vi "06.1 Injecting Errors.vi"() -> ()   [LabVIEW 2019]
uses:
  Support Files/02.4 DAQmx Configuration Cluster.ctl
  Support Files/03.2 States.ctl
  Support Files/03.2 State Machine Data.ctl
  <vilib>/DAQmx/write.llb/DAQmx Write (Analog DBL 1Chan 1Samp).vi
  <vilib>/Utility/file.llb/Write Delimited Spreadsheet (string).vi
  <vilib>/Utility/file.llb/Write Delimited Spreadsheet (DBL).vi
  <vilib>/DAQmx/create/channels.llb/DAQmx Create Channel (AO-Voltage-Basic).vi
  <vilib>/DAQmx/miscellaneous.llb/DAQmx Fill In Error Info.vi
panel:
  in  "DAQmx Configuration Cluster":T1={"Desired Sample Rate (Hz)"=-1.0, "sample mode"=10178, "Minimum value"=-1.0, "Maximum value"=-1.0, "Physical Channel"="", "units"=10143, "thermocouple type"=10072, "Samples per Channel"=0} {"thermocouple type" items=["J"=10072, "K"=10073, "N"=10077, "R"=10082, "S"=10085, "T"=10086, "B"=10047, "E"=10055]; "units" items=["Deg C"=10143, "Deg F"=10144, "Kelvins"=10325, "Deg R"=10145, "From Custom Scale"=10065]; "sample mode" items=["Finite Samples"=10178, "Continuous Samples"=10123, "Hardware Timed Single Point"=12522]}
  in  "Threshold (RMS)":dbl
  in  "Generate Stimulus":bool
  in  "Stop":bool
  in  "Clear":bool
  in  "Acquire":bool
  out "Graph":dbl[][](graph)
  out "Thershold Exceeded?":bool
  out "RMS Result per Channel":dbl[](array[numeric])
  # "ANALYSIS"
  # "EVENTS"
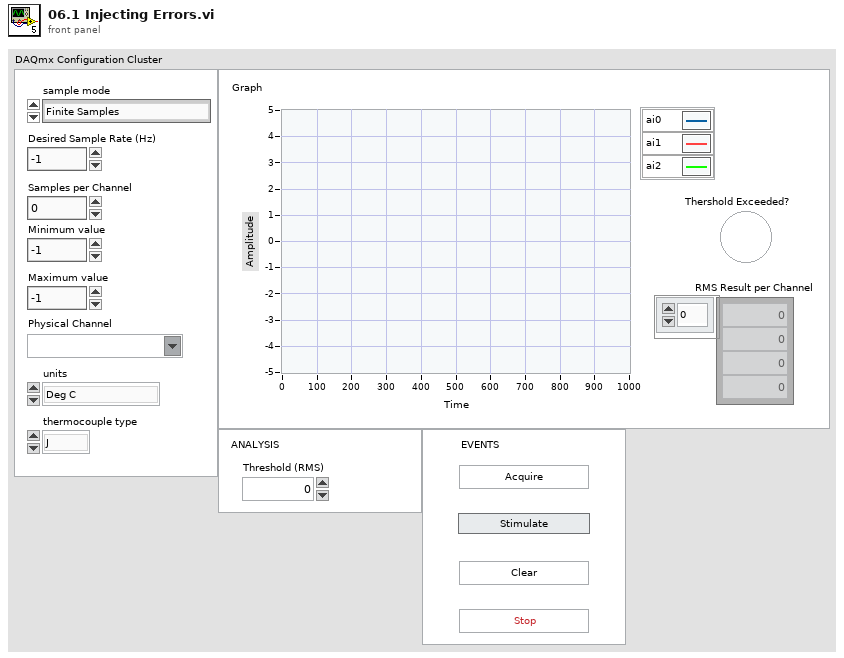
[diagram p1: front panel]
types:
  T1 = typedef "02.4 DAQmx Configuration Cluster.ctl" = cluster{"Desired Sample Rate (Hz)":dbl, "sample mode":i32, "Minimum value":dbl, "Maximum value":dbl, "Physical Channel":tag, "units":i32, "thermocouple type":i32, "Samples per Channel":i32}
  T2 = typedef "03.2 State Machine Data.ctl" = cluster{"Acquisition Data":dbl[][], "Stimulus?":bool}
  T3 = typedef "03.2 States.ctl" = enum16{"Initialize", "Update UI", "Update Stimulus", "Wait for event", "Acquire", "Analyze", "Log", "Clear", "Shutdown"}
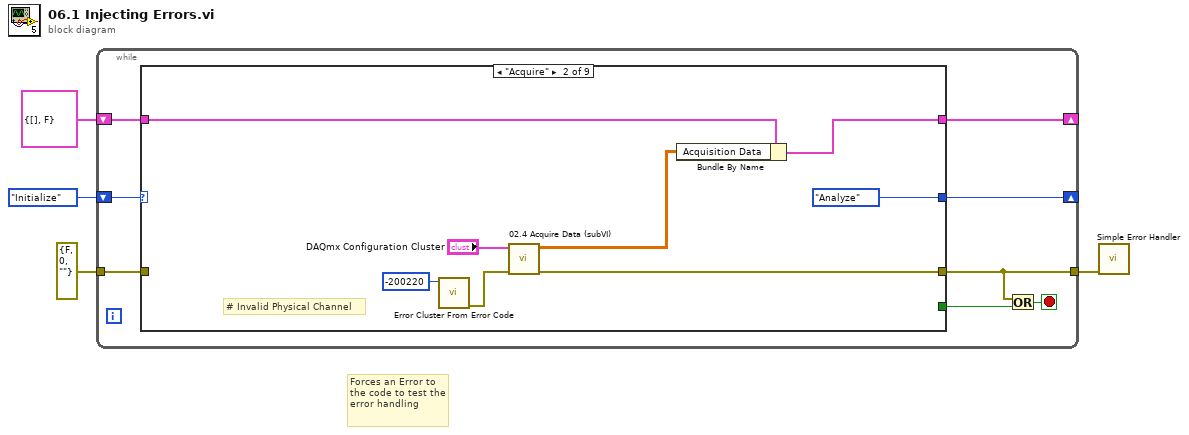
[diagram p0: block diagram]
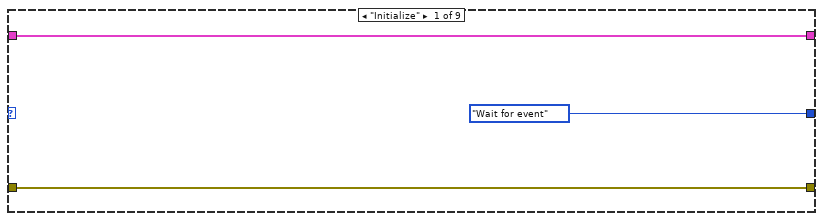
[diagram p2: hidden frame]
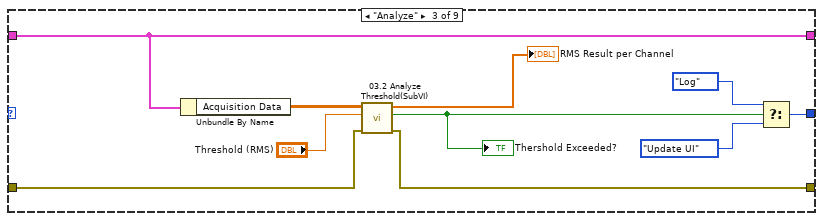
[diagram p3: hidden frame]
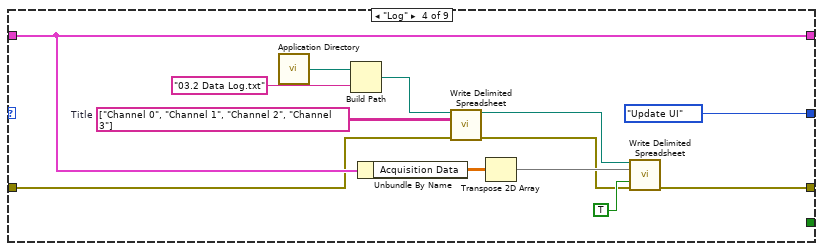
[diagram p4: hidden frame]
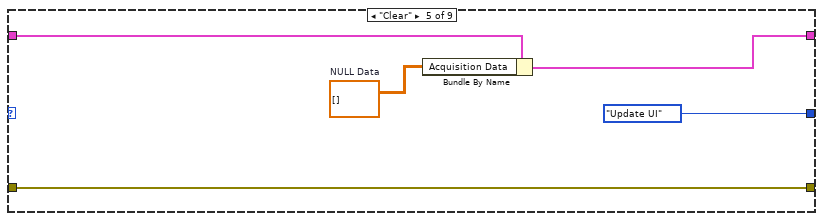
[diagram p5: hidden frame]
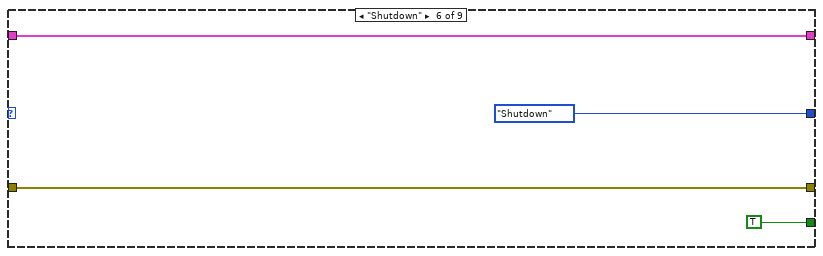
[diagram p6: hidden frame]
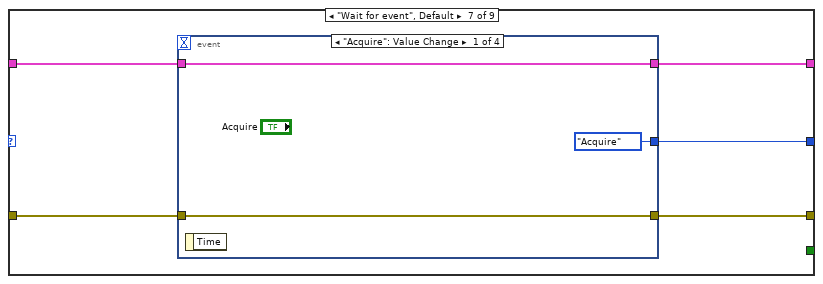
[diagram p7: hidden frame]
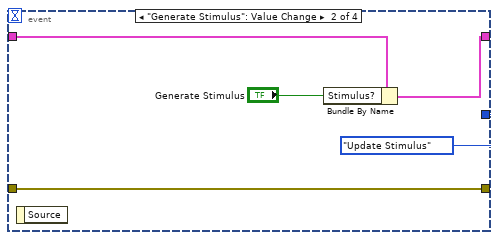
[diagram p8: hidden frame]
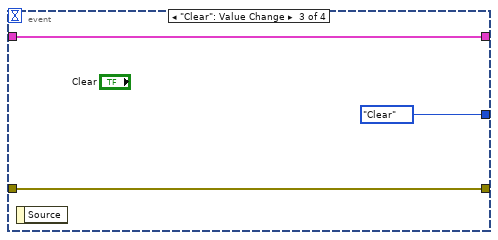
[diagram p9: hidden frame]
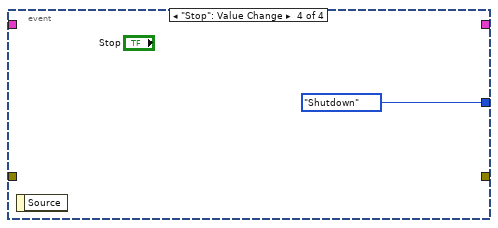
[diagram p10: hidden frame]
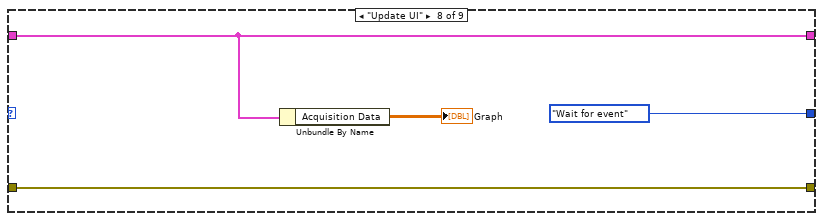
[diagram p11: hidden frame]
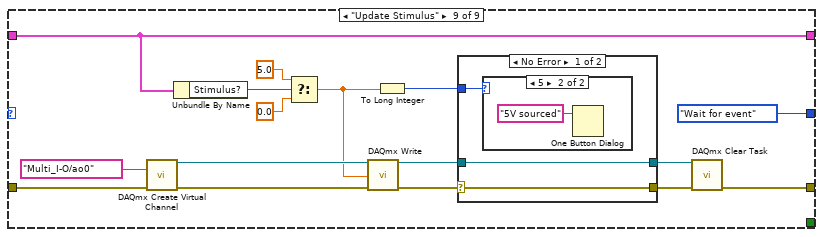
[diagram p12: hidden frame]
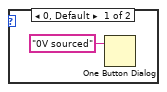
[diagram p13: hidden frame]
diagram:
  # "Forces an Error to the code to test the error handling"
  n1 = while {
    shift-right: [w11] -> _
    shift-left: 03.2_States."Initialize" ("State") -> [w12]
    tunnel: errorcluster {"status"=FALSE, "code"=0, "source"=""} ("error constant") -> [w10]
    tunnel: [w8] -> w2
    shift-right: [w7] -> _
    shift-left: T2 {"Acquisition Data"=[], "Stimulus?"=FALSE} -> [w6]
    stop <- w9 stop-if-true
    n2 = case shown="\"Acquire\"" w12 {
      tunnel: [03.2_States."Wait for event" ("State") 03.2_States."Analyze" ("State") w32 03.2_States."Update UI" ("State") 03.2_States."Update UI" ("State") 03.2_States."Shutdown" ("State") w60 03.2_States."Wait for event" ("State") 03.2_States."Wait for event" ("State")] -> w11
      tunnel: [w14 w20 w27 w44 w47 w53 w59 w74 w81] -> w8
      tunnel: w10 -> [w14 _ w28 w34 w47 w53 w58 w74 w92]
      tunnel: [w15 w22 w26 w42 w50 w54 w57 w76 w78] -> w7
      tunnel: w6 -> [w15 w23 w26 w42 w51 w54 w56 w76 w78]
      tunnel: [_ _ _ _ _ TRUE _ _ _] -> w5
      frame "Initialize" {
      }
      frame "Acquire" {
        # "# Invalid Physical Channel"
        n3 = call <vilib>:"Error Cluster From Error Code.vi"("error code (0)"=-200220) -> ("error out"=w17:errorcluster)  [unwired: 8 in]
        n4 = call "02.4 Acquire Data (subVI).vi"("Error In"=w17, "DAQmx Configuration Cluster"="DAQmx Configuration Cluster") -> ("error out"=w20:errorcluster, "2D DBL"=w21:dbl[][])  [unwired: 8 in]
        n5 = Bundle By Name(cluster=w23, "Acquisition Data"=w21) -> (w22:T2)
      }
      frame "Analyze" {
        n6 = Unbundle By Name(w26) -> ("Acquisition Data"=w33:dbl[][])
        n7 = call "03.2 Analyze Threshold(SubVI).vi"("Error In"=w28, "Threshold (RMS)"="Threshold (RMS)", "Data"=w33) -> ("Error Out"=w27:errorcluster, "Threshold exceeded?"=w29:bool, "RMS Results per Channel"=→"RMS Result per Channel":dbl[])  [unwired: 6 in]
        "Thershold Exceeded?" <- w29
        n8 = Select(t=03.2_States."Log" ("State"), s=w29, f=03.2_States."Update UI" ("State")) -> (s? t:f=w32:T3)
      }
      frame "Log" {
        w36 = string[][] [["Channel 0", "Channel 1", "Channel 2", "Channel 3"]]  # Title
        n9 = call <vilib>:"Application Directory.vi"() -> ("Application Directory"=w46:path)
        n10 = Build Path(base path=w46, name or relative path="03.2 Data Log.txt") -> (appended path=w37:path)
        n11 = Unbundle By Name(w42) -> ("Acquisition Data"=w41:dbl[][])
        n12 = call-poly <vilib>:"Write Delimited Spreadsheet.vi"("file path (dialog if empty)"=w37, "2D data"=w36, "error in (no error)"=w34) -> ("new file path (Not A Path if cancelled)"=w39:path, "error out"=w35:errorcluster)  [unwired: 11 in]
        n13 = Transpose 2D Array(2D array=w41) -> (transposed array=w40:dbl[][])
        n14 = call-poly <vilib>:"Write Delimited Spreadsheet.vi"("file path (dialog if empty)"=w39, "2D data"=w40, "append to file? (new file:F)"=TRUE, "error in (no error)"=w35) -> ("error out"=w44:errorcluster)  [unwired: 10 in, 1 out]
      }
      frame "Clear" {
        w49 = dbl[][] []  # NULL Data
        n15 = Bundle By Name(cluster=w51, "Acquisition Data"=w49) -> (w50:T2)
      }
      frame "Shutdown" {
      }
      frame "Wait for event", Default {
        n16 = event shown="[0] \"Acquire\": Value Change" {
          selector: _ -> [_ _ _ _]
          dyn-events: _ -> [_ _ _ _]
          timeout: _ -> [_ _ _ _]
          tunnel: [03.2_States."Acquire" ("State") 03.2_States."Update Stimulus" ("State") 03.2_States."Clear" ("State") 03.2_States."Shutdown" ("State")] -> w60
          tunnel: [w62 w64 w69 _] -> w59
          tunnel: w58 -> [w62 w64 w69 _]
          tunnel: [w61 w66 w71 _] -> w57
          tunnel: w56 -> [w61 w68 w71 _]
          event "Acquire": Value Change {
            n17 = event-data() -> ()  [unwired: 1 in, 1 out]
          }
          event "Generate Stimulus": Value Change {
            n18 = event-data() -> ()  [unwired: 1 in, 1 out]
            n19 = Bundle By Name(cluster=w68, "Stimulus?"="Generate Stimulus") -> (w66:T2)
          }
          event "Clear": Value Change {
            n20 = event-data() -> ()  [unwired: 1 in, 1 out]
          }
          event "Stop": Value Change {
            n21 = event-data() -> ()  [unwired: 1 in, 1 out]
          }
        }
      }
      frame "Update UI" {
        n22 = Unbundle By Name(w76) -> ("Acquisition Data"=→"Graph":dbl[][])
      }
      frame "Update Stimulus" {
        n23 = call-poly <vilib>:"DAQmx Create Virtual Channel.vi"("physical channels"=tag "Multi_I-O/ao0", "error in"=w92) -> ("task out"=w90:refnum<k21>, "error out"=w91:errorcluster)  [unwired: 12 in]
        n24 = Unbundle By Name(w78) -> ("Stimulus?"=w89:bool)
        n25 = Select(t=5.0, s=w89, f=0.0) -> (s? t:f=w86:dbl)
        n26 = call-poly <vilib>:"DAQmx Write.vi"("task/channels in"=w90, "data"=w86, "error in"=w91) -> ("task out"=w84:refnum<k21>, "error out"=w85:errorcluster)  [unwired: 10 in, 1 out]
        n27 = To Long Integer(number=w86) -> (32bit integer=w79:i32)
        n28 = case shown="No Error" w85 {
          selector: w85 -> [w95 w98]
          tunnel: w84 -> [w94 w99]
          tunnel: [w95 w98] -> w83
          tunnel: [w94 w99] -> w82
          tunnel: w79 -> [w93 _]
          frame No Error {
            n29 = case shown="5" w93 {
              frame 0, Default {
                n30 = One Button Dialog(message="0V sourced") -> ()  [unwired: 1 in, 1 out]
              }
              frame 5 {
                n31 = One Button Dialog(message="5V sourced") -> ()  [unwired: 1 in, 1 out]
              }
            }
          }
          frame Error {
          }
        }
        n32 = call <vilib>:"DAQmx Clear Task.vi"("task in"=w82, "error in"=w83) -> ("error out"=w81:errorcluster)  [unwired: 13 in]
      }
    }
    n33 = Or(x=w8, y=w5) -> (x .or. y?=w9:bool)
  }
  n34 = call <vilib>:"Simple Error Handler.vi"("error in (no error)"=w2) -> ()  [unwired: 4 in, 5 out]
